vi "Read CSV.vi"(8 "error in (no error)":errorcluster, 11 "Path":path) -> (0 "error out":errorcluster, 2 "first row":dbl[](array[numeric]) format="%0.3f", 3 "all rows":dbl[][](array[numeric]) format="%0.3f")   [LabVIEW 2013]
uses:
  <vilib>/Utility/file.llb/Read From Spreadsheet File (DBL).vi
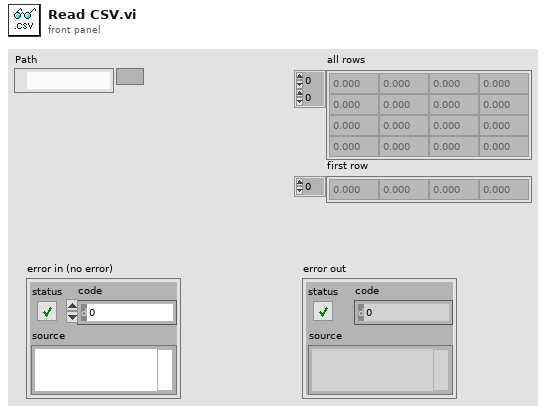
[diagram p1: front panel]
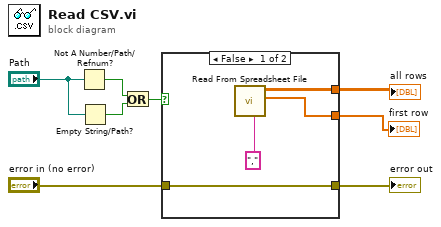
[diagram p0: block diagram]
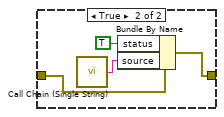
[diagram p2: hidden frame]
diagram:
  n1 = Not A Number/Path/Refnum?(number/path/refnum="Path") -> (NaN/Path/Refnum?=w8:bool)
  n2 = Empty String/Path?(string/path="Path") -> (empty?=w7:bool)
  n3 = Or(x=w8, y=w7) -> (x .or. y?=w5:bool)
  n4 = case shown="False" w5 {
    tunnel: "error in (no error)" -> [w11 w16]
    tunnel: [w11 w13] -> w3
    tunnel: [w10 _] -> w2
    tunnel: [w9 _] -> w1
    frame False {
      n5 = call-poly <vilib>:"Read From Spreadsheet File.vi"("delimiter (\\t)"="," ("delimiter (\\t)")) -> ("first row"=w9:dbl[], "all rows"=w10:dbl[][])  [unwired: 6 in, 3 out]
    }
    frame True {
      n6 = call "Call Chain (Single String).vi"() -> ("Call Chain"=w14:string)
      n7 = Bundle By Name(cluster=w16, "status"=TRUE, "source"=w14) -> (w13:errorcluster)
    }
  }
  "error out" <- w3
  "all rows" <- w2
  "first row" <- w1
